vi "Create.vi"(8 "error in (no error)":errorcluster) -> (0 "error out":errorcluster, 3 "Identical Inputs Comparator":refnum<class "Identical Inputs Comparator.lvclass">)   [LabVIEW 2020, in "Identical Inputs Comparator.lvclass"]
uses:
  Identical Inputs Comparator.lvclass
  Identical Inputs Comparator.lvclass/Identical Inputs Comparator.ctl
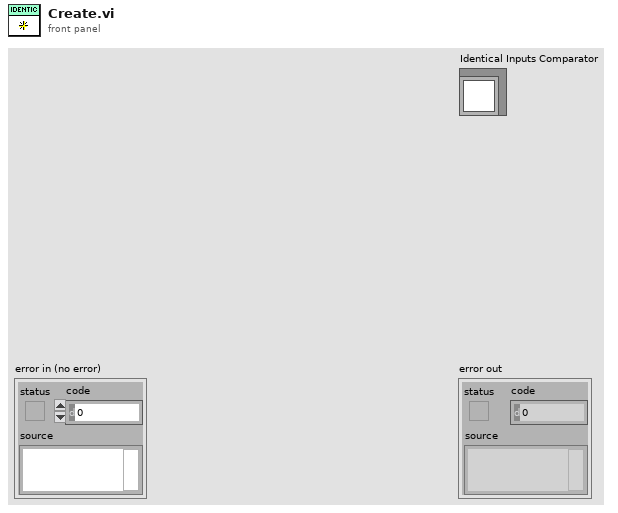
[diagram p1: front panel]
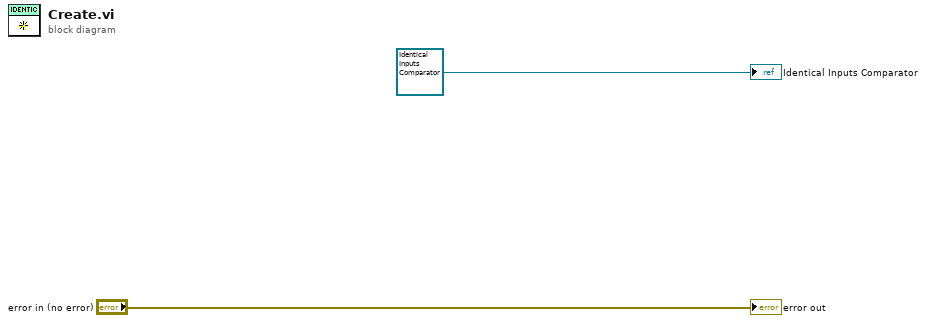
[diagram p0: block diagram]
diagram:
  "error out" <- "error in (no error)"
  "Identical Inputs Comparator" <- refnum<class "Identical Inputs Comparator.lvclass"> refnum ("Identical Inputs Comparator")
